vi "8502_List.vi"() -> ()   [LabVIEW 2016]
uses:
  <instrlib>/BK Precision 85XX Series/BK Precision 85XX Series.lvlib
panel:
  out "error out":errorcluster
  out "Step Timing":dbl
  out "Step Value":dbl
  out "List Step Number":dbl
  out "VISA resource name out":refnum<visa-resource-name>
  out "Mode of Operation":u8
  out "Number of Steps":u16
  out "List Operation":u8
  in  "Communication Address (0)":u8 max=254 format="%x"
  in  "Serial Configuration":T1={"Baud Rate"=9600, "Parity"=0, "Data Bits"=8, "Stop Bits"=10} {"Stop Bits" items=["1.0"=10]; "Data Bits" items=["8"=8]; "Parity" items=["None", "Odd", "Even"]; "Baud Rate" items=["4800"=4800, "9600"=9600, "19200"=19200, "38400"=38400]}
  in  "VISA resource name":refnum<visa-resource-name>
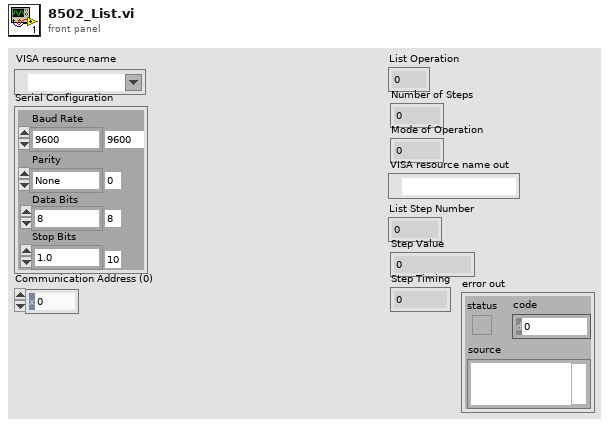
[diagram p1: front panel]
types:
  T1 = cluster{"Baud Rate":u32, "Parity":u16, "Data Bits":u16, "Stop Bits":u16}
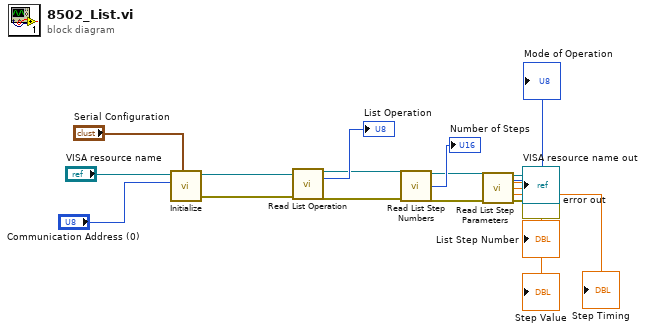
[diagram p0: block diagram]
diagram:
  n1 = call <instrlib>:"Initialize.vi"("Serial Configuration"="Serial Configuration", "Communication Address (0)"="Communication Address (0)", "VISA resource name"="VISA resource name") -> ("error out"=w13:errorcluster, "VISA resource name out"=w14:refnum<visa-resource-name>)  [unwired: 7 in]
  n2 = call <instrlib>:"Read List Operation.vi"("VISA resource name"=w14, "error in (no error)"=w13) -> ("VISA resource name out"=w11:refnum<visa-resource-name>, "List Operation"=→"List Operation":u8, "error out"=w10:errorcluster)  [unwired: 10 in, 1 out]
  n3 = call <instrlib>:"Read List Step Numbers.vi"("VISA resource name"=w11, "error in (no error)"=w10) -> ("VISA resource name out"=w8:refnum<visa-resource-name>, "Number of Steps"=→"Number of Steps":u16, "error out"=w7:errorcluster)  [unwired: 11 in]
  n4 = call <instrlib>:"Read List Step Parameters.vi"("VISA resource name"=w8, "error in (no error)"=w7) -> ("Mode of Operation"=→"Mode of Operation":u8, "VISA resource name out"=→"VISA resource name out":refnum<visa-resource-name>, "List Step Number"=→"List Step Number":dbl, "Step Value"=→"Step Value":dbl, "Step Timing"=→"Step Timing":dbl, "error out"=→"error out":errorcluster)  [unwired: 8 in]
